vi "GetElementOfAnalogWaveform.vi"(8 "error in (no error)":errorcluster, 10 "index":i32, 11 "Oscilloscope in":refnum<class "Oscilloscope.lvclass">) -> (0 "error out":errorcluster, 2 "Analog Waveforms":waveform(dbl), 3 "Oscilloscope out":refnum<class "Oscilloscope.lvclass">)   [LabVIEW 2020, in "Oscilloscope.lvclass"]
uses:
  Oscilloscope.lvclass
  Oscilloscope.lvclass/Oscilloscope.ctl
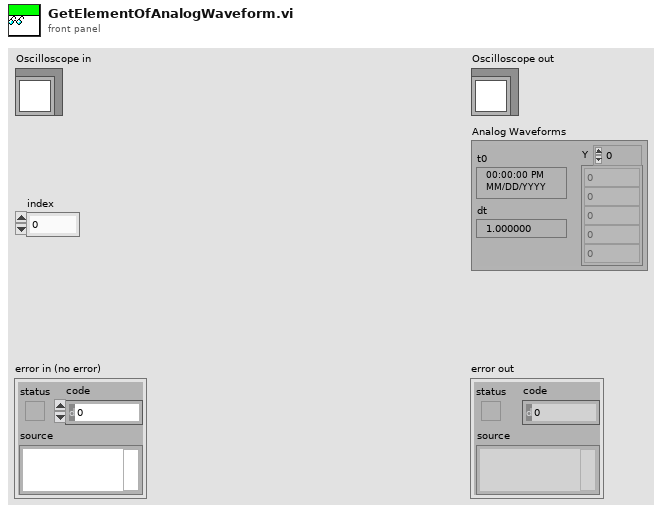
[diagram p1: front panel]
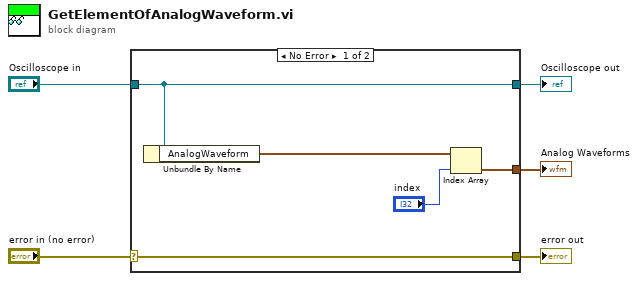
[diagram p0: block diagram]
diagram:
  n1 = case shown="No Error" "error in (no error)" {
    selector: "error in (no error)" -> [w10 w11]
    tunnel: [w10 w11] -> w4
    tunnel: [w9 w12] -> w2
    tunnel: "Oscilloscope in" -> [w9 w12]
    tunnel: [w6 _] -> w1
    frame No Error {
      n2 = Unbundle By Name(w9) -> ("AnalogWaveform"=w8:waveform(dbl)[])
      n3 = Index Array(array=w8, index="index") -> (element=w6:waveform(dbl))
    }
    frame Error {
    }
  }
  "error out" <- w4
  "Oscilloscope out" <- w2
  "Analog Waveforms" <- w1
